vi "Responce Parse.vi"(11 "Responce":string) -> (1 "Payload":string, 2 "Command":string, 3 "Address":u8, 4 "Error Code":i8, 5 "OK":bool, 6 "Error?":bool, 7 "Checksum OK":bool)   [LabVIEW 2017, in "Samwontech TEMP2xxx.lvlib"]
uses:
  <instrlib>/Samwontech TEMP2xxx/Samwontech TEMP2xxx.lvlib
panel:
  out "Probe: Calculated \nSUM (byte)":u8 format="%.0x"
  out "Probe: Responce SUM":string
  out "Probe: Responce without SUM":string
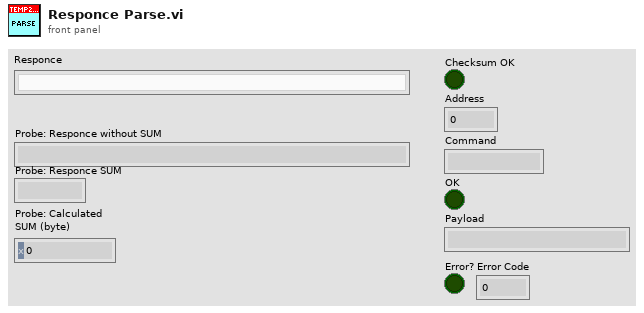
[diagram p1: front panel]
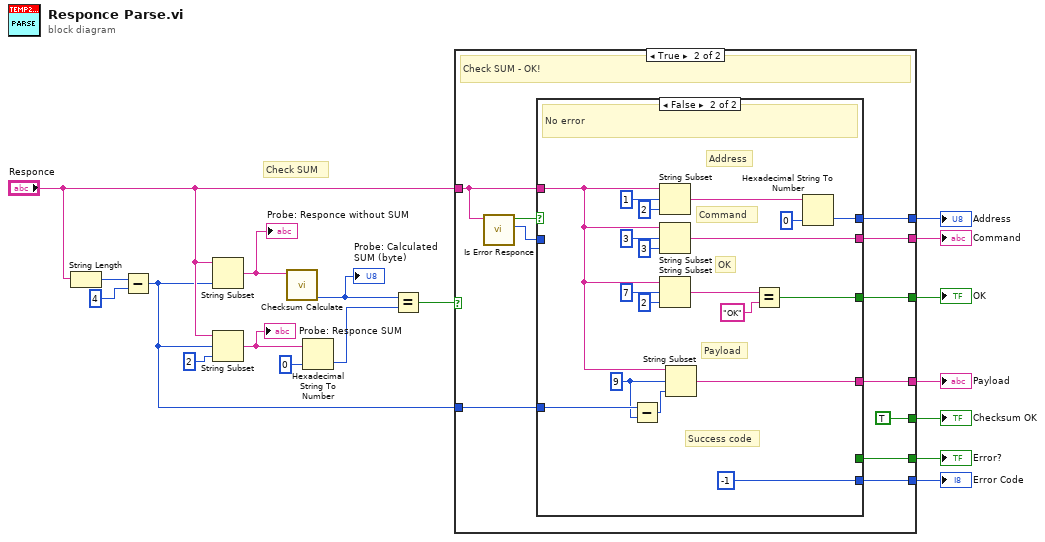
[diagram p0: block diagram]
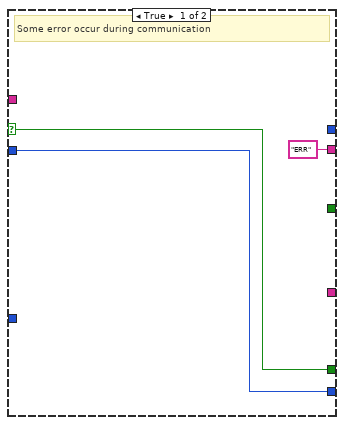
[diagram p3: hidden frame]
diagram:
  # "Check SUM"
  n1 = String Length(string="Responce") -> (length=w18:i32)
  n2 = Subtract(x=w18, y=4) -> (x-y=w7:i32)
  n3 = String Subset(string="Responce", length (rest)=w7) -> (substring=w15:string)  [unwired: 1 in]
  "Probe: Responce without SUM" <- w15
  n4 = String Subset(string="Responce", offset (0)=w7, length (rest)=2 ("length (rest)")) -> (substring=w14:string)
  "Probe: Responce SUM" <- w14
  n5 = call <instrlib>:"Checksum Calculate.vi"("Command in"=w15) -> ("Checksum (byte)"=w13:u8)  [unwired: 7 in, 3 out]
  "Probe: Calculated \nSUM (byte)" <- w13
  n6 = Hexadecimal String To Number(string=w14, default (0uL)=u8 0) -> (number=w12:u8)  [unwired: 1 in, 1 out]
  n7 = Equal?(x=w13, y=w12) -> (x = y?=w11:bool)
  n8 = case shown="True" w11 {
    tunnel: "Responce" -> [_ w25]
    tunnel: [_ w26] -> w9
    tunnel: [_ w29] -> w6
    tunnel: w7 -> [_ w28]
    tunnel: [_ TRUE] -> w5
    tunnel: [_ w23] -> w4
    tunnel: [_ w22] -> w3
    tunnel: [_ w20] -> w2
    tunnel: [_ w19] -> w1
    frame False {
    }
    frame True {
      # "Check SUM - OK!"
      n9 = call <instrlib>:"Is Error Responce.vi"("Responce"=w25) -> ("Error Code"=w21:i8, "Error?"=w24:bool)  [unwired: 9 in]
      n10 = case shown="False" w24 {
        selector: w24 -> [w31 _]
        tunnel: [_ w47] -> w29
        tunnel: w28 -> [_ w46]
        tunnel: ["ERR" ("Responce") w41] -> w26
        tunnel: w25 -> [_ w40]
        tunnel: [_ w37] -> w23
        tunnel: [_ w34] -> w22
        tunnel: w21 -> [w30 _]
        tunnel: [w31 _] -> w20
        tunnel: [w30 i8 -1 ("Error Code")] -> w19
        frame True {
          # "Some error occur during communication"
        }
        frame False {
          w45 = 9 ("length (rest)")
          # "Success code"
          # "OK"
          # "Payload"
          # "Command"
          # "Address"
          # "No error"
          n11 = Subtract(x=w46, y=w45) -> (x-y=w44:i32)
          n12 = String Subset(string=w40, offset (0)=1 ("length (rest)"), length (rest)=2 ("length (rest)")) -> (substring=w35:string)
          n13 = String Subset(string=w40, offset (0)=3 ("length (rest)"), length (rest)=3 ("length (rest)")) -> (substring=w41:string)
          n14 = String Subset(string=w40, offset (0)=7 ("length (rest)"), length (rest)=2 ("length (rest)")) -> (substring=w38:string)
          n15 = String Subset(string=w40, offset (0)=w45, length (rest)=w44) -> (substring=w47:string)
          n16 = Equal?(x=w38, y="OK") -> (x = y?=w37:bool)
          n17 = Hexadecimal String To Number(string=w35, default (0uL)=u8 0) -> (number=w34:u8)  [unwired: 1 in, 1 out]
        }
      }
    }
  }
  "Address" <- w3
  "Command" <- w9
  "Payload" <- w6
  "Checksum OK" <- w5
  "OK" <- w4
  "Error?" <- w2
  "Error Code" <- w1
